vi "HCC Cluster Arrays ReadWrite.vi"(0 "Array Label":string(combo)="Aisle1", 1 "Write?":bool, 5 "configuration file path":path=path "C:/data/Wilt Backup.ini", 7 "Array Dryers In":T1[](array[typedef]) {"Unit Type" items=["", "Viper", "Hawk", "Other"]; "Current" format="%.2f"; "Day Cycle Count" format="%04d"}, 11 "error in (no error)":errorcluster) -> (8 "Array Dryers Out":T1[](array[typedef]) {"Unit Type" items=["", "Viper", "Hawk", "Other"]; "Current" format="%.2f"; "Day Cycle Count" format="%04d"}, 15 "error out":errorcluster)   [LabVIEW 2012]
uses:
  <vilib>/Utility/VariantDataType/Type.ctl
  Nufi/Newfi LDN/Washer.ctl
  Nufi/Newfi LDN/Washer Details.ctl
  Nufi/Newfi LDN/Unit Type.ctl
  <vilib>/Utility/config.llb/Write Key (Double).vi
  <vilib>/Utility/config.llb/Write Key (String).vi
  <vilib>/Utility/config.llb/Write Key (Path).vi
  <vilib>/Utility/config.llb/Write Key (I32).vi
  <vilib>/Utility/config.llb/Write Key (U32).vi
  <vilib>/Utility/config.llb/Write Key (Boolean).vi
  <vilib>/Utility/config.llb/Read Key (Double).vi
  <vilib>/Utility/config.llb/Read Key (String).vi
  <vilib>/Utility/config.llb/Read Key (Path).vi
  <vilib>/Utility/config.llb/Read Key (I32).vi
  <vilib>/Utility/config.llb/Read Key (U32).vi
  <vilib>/Utility/config.llb/Read Key (Boolean).vi
  <vilib>/Utility/config.llb/NI_LVConfig.lvlib
  <vilib>/Utility/VariantDataType/VariantType.lvlib
panel:
  out "Label.Text 2":string
  out "Local Control?":bool
  in  "Array Dryers Display":T1[](array[typedef]) {"Unit Type" items=["", "Viper", "Hawk", "Other"]; "Current" format="%.2f"; "Day Cycle Count" format="%04d"}
  out "value":string
  in  "Dryer Variable":T1 {"Unit Type" items=["", "Viper", "Hawk", "Other"]; "Current" format="%.2f"; "Day Cycle Count" format="%04d"}
  out "String array out":string="[1,23-2-3]\n[4-3,22-2]\n[3-4,01-8]\n[0-7-6,66]"
  out "Label.Text":string
  out "Type Enum":T4
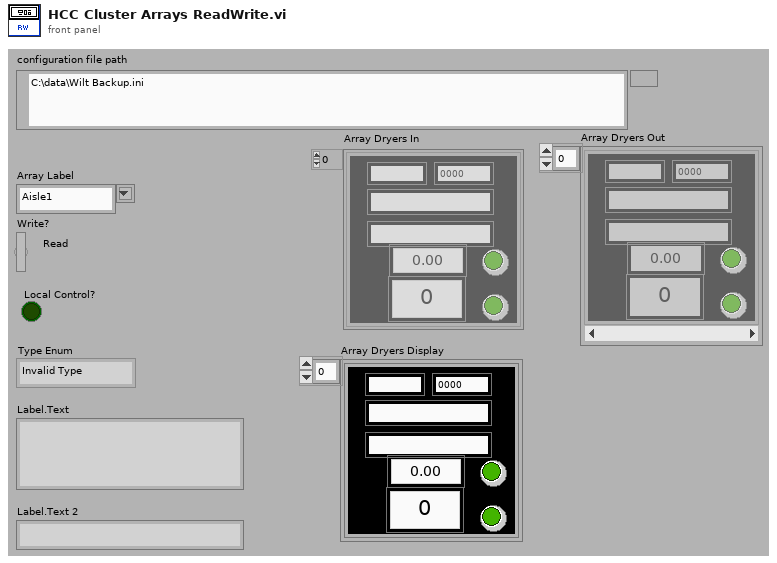
[diagram p1: front panel]
types:
  T1 = typedef "Washer.ctl" = cluster{"Serial Number":string, "Day Cycle Count":i32, "Station Label":string, "Status Color":u32, "Current Run Start Time":dbl, "Audit Alert":bool, "Washer Details":T2, "Board ID":string, "Boolean":bool, "RPM":u32, "Current":dbl, "Current Path":path, "Saving":bool, "Unit Type":T3}
  T2 = typedef "Washer Details.ctl" = cluster{"Cycle Count":string, "Status":string, "Notes":string, "Lab ID":string, "Total Time On":string, "TR Number":string}
  T3 = typedef "Unit Type.ctl" = u32
  T4 = typedef "VariantType.lvlib/Type.ctl" = enum8{"Invalid Type", "Void", "I8", "I16", "I32", "I64", "U8", "U16", "U32", "U64", "Single Float", "Double Float", "Extended Float", "Single Complex", "Double Complex", "Extended Complex", "Enum U8", "Enum U16", "Enum U32", "Enum U64", "Single Float With Unit", "Double Float With Unit", "Extended Float With Unit", "Single Complex with Unit", "Double Complex with Unit", "Extended Complex with Unit", "Boolean", "String", "Path", "Picture", "Tag", "Array", "Cluster", "Variant", "LV Variant", "Waveform", "Timestamp", "Digital Waveform", "Digital Data", "ExpressData", "Refnum", "External Data", "VI", "Poly VI", "LabVIEW Class Instance", "Fixed Point"}
  T5 = typedef "NI_LVConfig.lvlib/Config Data RefNum.ctl" = refnum<k1>
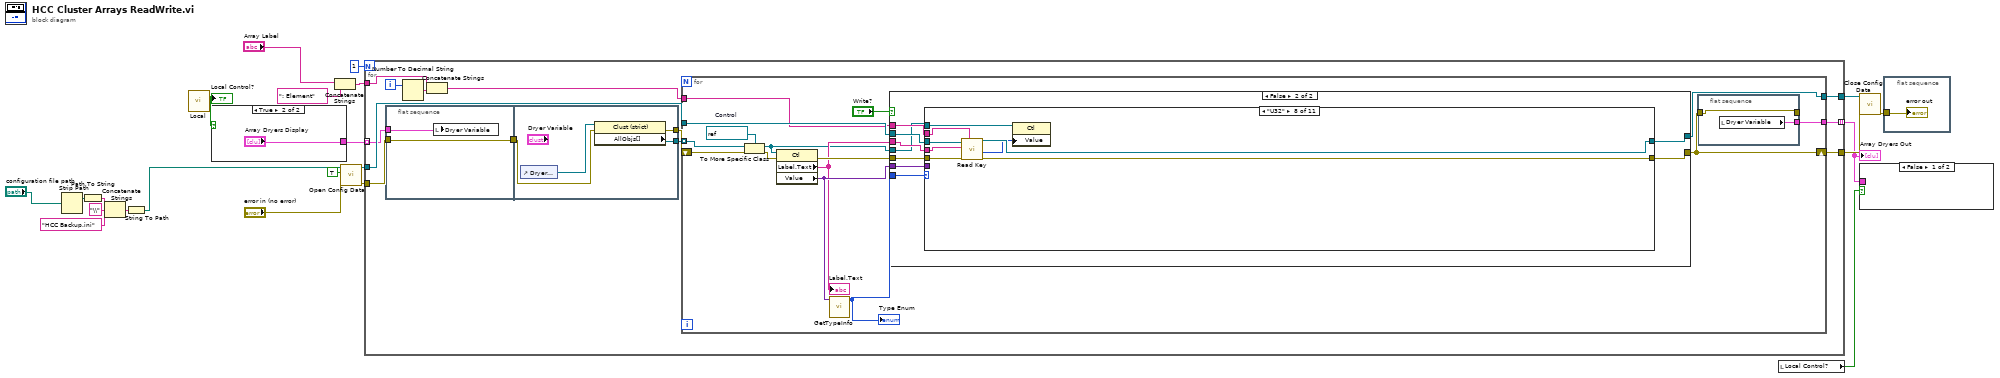
[diagram p0: block diagram]
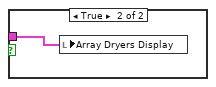
[diagram p2: hidden frame]
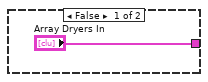
[diagram p3: hidden frame]
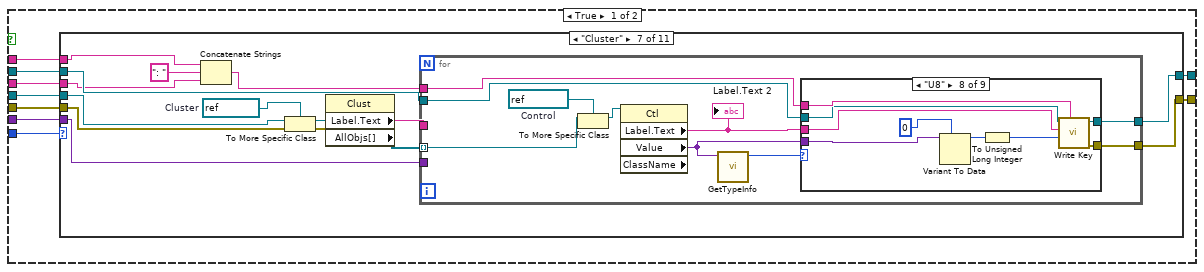
[diagram p4: hidden frame]
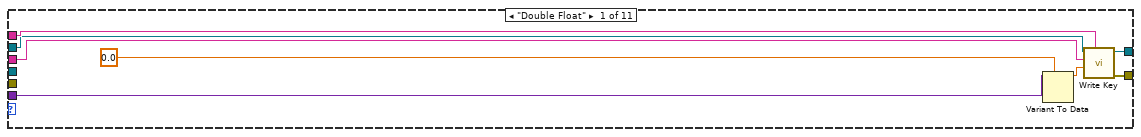
[diagram p5: hidden frame]
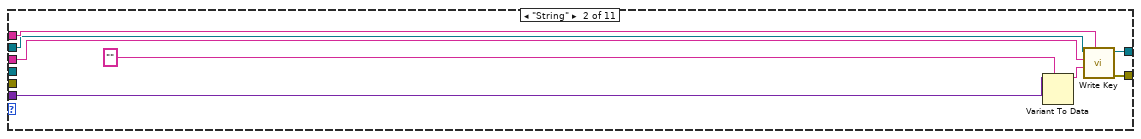
[diagram p6: hidden frame]
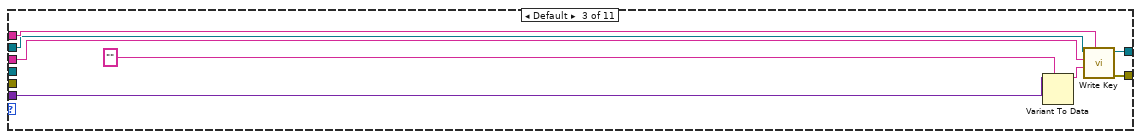
[diagram p7: hidden frame]
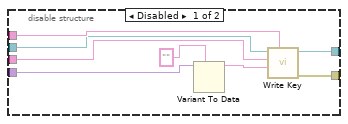
[diagram p9: hidden frame]
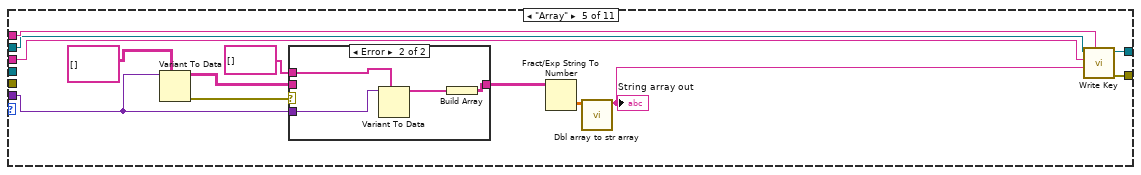
[diagram p10: hidden frame]
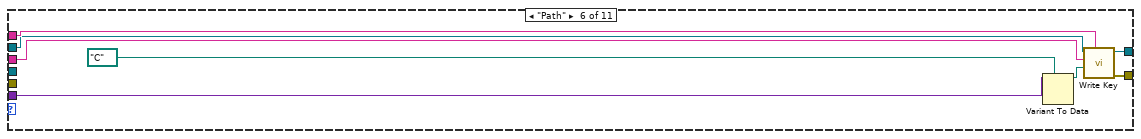
[diagram p12: hidden frame]
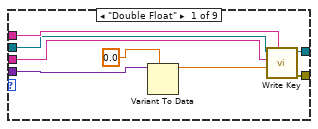
[diagram p13: hidden frame]
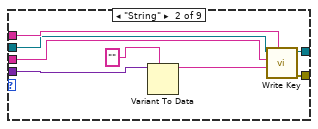
[diagram p14: hidden frame]
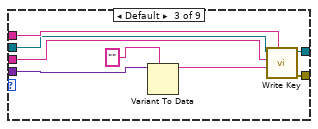
[diagram p15: hidden frame]
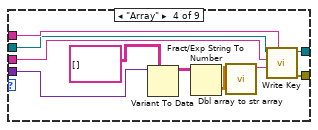
[diagram p16: hidden frame]
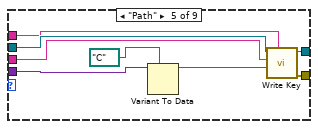
[diagram p17: hidden frame]
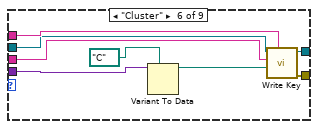
[diagram p18: hidden frame]
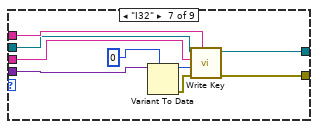
[diagram p19: hidden frame]
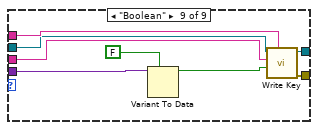
[diagram p20: hidden frame]
diagram:
  n1 = Strip Path(path="configuration file path") -> (stripped path=w5:path)  [unwired: 1 out]
  n2 = Path To String(path=w5) -> (string=w4:string)
  n3 = Concatenate Strings(w4, "\\" ("string"), "HCC Backup.ini" ("string")) -> (w8:string)
  n4 = String To Path(string=w8) -> (path=w2:path)
  n5 = call "Local.vi"() -> ("Local?"=w9:bool)  [unwired: 11 in]
  "Local Control?" <- w9
  n6 = case shown="True" w9 {
    tunnel: ["Array Dryers In" "Array Dryers Display"] -> w11
    frame False {
    }
    frame True {
    }
  }
  n7 = Concatenate Strings("Array Label", ": Element" ("string")) -> (w16:string)
  n8 = call <vilib>:"Open Config Data.vi"("error in (no error)"="error in (no error)", "create file if necessary (T)"=TRUE, "configuration file path"=w2) -> ("error out"=w19:errorcluster, "refnum"=w21:T5)  [unwired: 6 in, 1 out]
  n9 = for {
    N: 1 -> [_]
    tunnel: w19 -> [w36]
    tunnel: w11 -> [w32] mode=indexing
    tunnel: w21 -> [w34]
    tunnel: w16 -> [w30]
    tunnel: [w27] -> w14
    tunnel: [w26] -> w13
    tunnel: [w25] -> w12 mode=indexing
    i -> [w28]
    n10 = flat-sequence {
      tunnel: w36 -> [w39]
      tunnel: [w39] -> w33
      tunnel: w32 -> [w38]
      tunnel: [w43] -> w37
      tunnel: [w41] -> w35
      tunnel: w33 -> [w42]
      frame #0 {
        n11 = local write "Dryer Variable"(w38) -> ()
      }
      frame #1 {
        n12 = control-ref of="Dryer Variable"() -> (w40:refnum<vi>)
        n13 = property class="Clust (strict)"(reference=w40, error in=w42) -> (error out=w41:errorcluster, "AllObjs[]"=w43:refnum<vi>[])  [unwired: 1 out]
      }
    }
    n14 = Number To Decimal String(number=w28) -> (decimal integer string=w31:string)  [unwired: 1 in]
    n15 = Concatenate Strings(w30, w31) -> (w29:string)
    n16 = for {
      tunnel: w37 -> [w58] mode=indexing
      tunnel: w34 -> [w56]
      tunnel: [w55] -> w26
      shift-right: [w46] -> w27
      shift-left: w35 -> [w54]
      tunnel: w29 -> [w47]
      tunnel: [w45] -> w25
      w57 = refnum<vi> refnum  # Control
      n17 = To More Specific Class(target class=w57, reference=w58, error in=w54) -> (specific class reference=w44:refnum<vi>, error out=w49:errorcluster)
      n18 = property class="Ctl"(reference=w44, error in=w49) -> (error out=w50:errorcluster, "Label.Text"=w48:string, "Value"=w51:variant)  [unwired: 1 out]
      "Label.Text" <- w48
      n19 = call <vilib>:"GetTypeInfo.vi"("Variant"=w51) -> ("Type Enum"=w52:T4)  [unwired: 6 in, 4 out]
      "Type Enum" <- w52
      n20 = case shown="False" "Write?" {
        tunnel: w47 -> [w69 w276]
        tunnel: w48 -> [w68 w275]
        tunnel: w51 -> [w67 w268]
        tunnel: w56 -> [w66 w274]
        tunnel: [w65 w273] -> w46
        tunnel: [w64 w272] -> w55
        tunnel: w44 -> [w61 w271]
        tunnel: w52 -> [w63 w270]
        tunnel: w50 -> [w62 w269]
        frame True {
          n21 = case shown="\"Cluster\"" w63 {
            tunnel: w69 -> [w77 w85 w93 w99 w120 w133 w136 w242 w250 w259 w267]
            tunnel: w68 -> [w76 w84 w92 w98 w119 w132 w135 w241 w249 w258 w266]
            tunnel: w67 -> [w75 w83 w91 w97 w109 w131 w144 w240 w248 w257 w265]
            tunnel: w66 -> [w74 w82 w90 w96 w118 w130 w138 w239 w247 w256 w264]
            tunnel: [w73 w81 w89 w95 w117 w129 w142 w238 w246 w255 w263] -> w65
            tunnel: [w72 w80 w88 w94 w116 w128 w143 w237 w245 w254 w262] -> w64
            tunnel: w62 -> [_ _ _ _ _ _ w145 _ _ _ _]
            tunnel: w61 -> [_ _ _ _ _ _ w140 _ _ _ _]
            frame "Double Float" {
              n22 = Variant To Data(type=0.0, Variant=w75) -> (data=w71:dbl)  [unwired: 1 in, 1 out]
              n23 = call-poly <vilib>:"Write Key.vi"("section"=w77, "value"=w71, "key"=w76, "refnum"=w74) -> ("error out"=w73:errorcluster, "refnum out"=w72:T5)  [unwired: 5 in, 1 out]
            }
            frame "String" {
              n24 = Variant To Data(type="" ("Label.Text"), Variant=w83) -> (data=w79:string)  [unwired: 1 in, 1 out]
              n25 = call-poly <vilib>:"Write Key.vi"("section"=w85, "value"=w79, "key"=w84, "refnum"=w82) -> ("error out"=w81:errorcluster, "refnum out"=w80:T5)  [unwired: 5 in, 1 out]
            }
            frame Default {
              n26 = Variant To Data(type="" ("Label.Text"), Variant=w91) -> (data=w87:string)  [unwired: 1 in, 1 out]
              n27 = call-poly <vilib>:"Write Key.vi"("section"=w93, "value"=w87, "key"=w92, "refnum"=w90) -> ("error out"=w89:errorcluster, "refnum out"=w88:T5)  [unwired: 5 in, 1 out]
            }
            frame "Void" {
              n28 = disable-structure shown="Enabled" {
                disable-tunnel: w99 -> [w107 _]
                disable-tunnel: w98 -> [w106 _]
                disable-tunnel: w97 -> [w105 _]
                disable-tunnel: w96 -> [w104 _]
                disable-tunnel: [w103 _] -> w95
                disable-tunnel: [w102 _] -> w94
                frame Disabled {
                  n29 = Variant To Data(type="" ("Label.Text"), Variant=w105) -> (data=w101:string)  [unwired: 1 in, 1 out]
                  n30 = call-poly <vilib>:"Write Key.vi"("section"=w107, "value"=w101, "key"=w106, "refnum"=w104) -> ("error out"=w103:errorcluster, "refnum out"=w102:T5)  [unwired: 5 in, 1 out]
                }
                frame Enabled {
                }
              }
            }
            frame "Array" {
              n31 = Variant To Data(type=string[][] [], Variant=w109) -> (data=w111:string[][], error out=w112:errorcluster)  [unwired: 1 in]
              n32 = case shown="Error" w112 {
                tunnel: [w121 w122] -> w110
                tunnel: w111 -> [w121 _]
                tunnel: w109 -> [_ w125]
                tunnel: string[] [] -> [_ w124]
                frame No Error {
                }
                frame Error {
                  n33 = Variant To Data(type=w124, Variant=w125) -> (data=w123:string[])  [unwired: 1 in, 1 out]
                  n34 = Build Array(w123) -> (w122:string[][])
                }
              }
              n35 = Fract/Exp String To Number(string=w110) -> (number=w114:dbl[][])  [unwired: 3 in, 1 out]
              n36 = call "Dbl array to str array.vi"("Array in"=w114) -> ("String array out"=w113:string)  [unwired: 9 in, 1 out]
              "String array out" <- w113
              n37 = call-poly <vilib>:"Write Key.vi"("section"=w120, "value"=w113, "key"=w119, "refnum"=w118) -> ("error out"=w117:errorcluster, "refnum out"=w116:T5)  [unwired: 5 in, 1 out]
            }
            frame "Path" {
              n38 = Variant To Data(type=path "C:/" ("configuration file path 2"), Variant=w131) -> (data=w127:path)  [unwired: 1 in, 1 out]
              n39 = call-poly <vilib>:"Write Key.vi"("section"=w133, "value"=w127, "key"=w132, "refnum"=w130) -> ("error out"=w129:errorcluster, "refnum out"=w128:T5)  [unwired: 5 in, 1 out]
            }
            frame "Cluster" {
              w148 = refnum<vi> refnum  # Cluster
              n40 = Concatenate Strings(w136, ": " ("string"), w135) -> (w137:string)
              n41 = To More Specific Class(target class=w148, reference=w140, error in=w145) -> (specific class reference=w147:refnum<vi>, error out=w146:errorcluster)
              n42 = property class="Clust"(reference=w147, error in=w146) -> ("Label.Text"=w141:string, "AllObjs[]"=w139:refnum<vi>[])  [unwired: 2 out]
              n43 = for {
                tunnel: w144 -> [_]
                tunnel: w137 -> [w158]
                tunnel: w139 -> [w153] mode=indexing
                tunnel: [w157] -> w143
                tunnel: [w156] -> w142
                tunnel: w141 -> [_]
                tunnel: w138 -> [w152]
                w155 = refnum<vi> refnum  # Control
                n44 = To More Specific Class(target class=w155, reference=w153) -> (specific class reference=w154:refnum<vi>)  [unwired: 1 in, 1 out]
                n45 = property class="Ctl" props=["Label", "Text", "Value", "ClassName"](reference=w154) -> ("Label.Text"=w149:string, "Value"=w150:variant)  [unwired: 1 in, 3 out]
                "Label.Text 2" <- w149
                n46 = call <vilib>:"GetTypeInfo.vi"("Variant"=w150) -> ("Type Enum"=w151:T4)  [unwired: 6 in, 4 out]
                n47 = case shown="\"U8\"" w151 {
                  tunnel: w158 -> [w166 w174 w182 w192 w194 w208 w217 w226 w234]
                  tunnel: w149 -> [w165 w173 w175 w191 w193 w207 w216 w225 w233]
                  tunnel: w150 -> [w164 w172 w181 w190 w200 w206 w215 w224 w232]
                  tunnel: w152 -> [w159 w167 w176 w183 w195 w201 w209 w218 w227]
                  tunnel: [w163 w171 w180 w189 w199 w205 w214 w223 w231] -> w156
                  tunnel: [w162 w170 w179 w188 w198 w204 w213 w222 w230] -> w157
                  frame "Double Float" {
                    n48 = Variant To Data(type=0.0, Variant=w164) -> (data=w160:dbl)  [unwired: 1 in, 1 out]
                    n49 = call-poly <vilib>:"Write Key.vi"("section"=w166, "value"=w160, "key"=w165, "refnum"=w159) -> ("error out"=w163:errorcluster, "refnum out"=w162:T5)  [unwired: 5 in, 1 out]
                  }
                  frame "String" {
                    n50 = Variant To Data(type="" ("Label.Text"), Variant=w172) -> (data=w168:string)  [unwired: 1 in, 1 out]
                    n51 = call-poly <vilib>:"Write Key.vi"("section"=w174, "value"=w168, "key"=w173, "refnum"=w167) -> ("error out"=w171:errorcluster, "refnum out"=w170:T5)  [unwired: 5 in, 1 out]
                  }
                  frame Default {
                    n52 = Variant To Data(type="" ("Label.Text"), Variant=w181) -> (data=w177:string)  [unwired: 1 in, 1 out]
                    n53 = call-poly <vilib>:"Write Key.vi"("section"=w182, "value"=w177, "key"=w175, "refnum"=w176) -> ("error out"=w180:errorcluster, "refnum out"=w179:T5)  [unwired: 5 in, 1 out]
                  }
                  frame "Array" {
                    n54 = Variant To Data(type=string[][] [], Variant=w190) -> (data=w186:string[][])  [unwired: 1 in, 1 out]
                    n55 = Fract/Exp String To Number(string=w186) -> (number=w185:dbl[][])  [unwired: 3 in, 1 out]
                    n56 = call "Dbl array to str array.vi"("Array in"=w185) -> ("String array out"=w184:string)  [unwired: 9 in, 1 out]
                    n57 = call-poly <vilib>:"Write Key.vi"("section"=w192, "value"=w184, "key"=w191, "refnum"=w183) -> ("error out"=w189:errorcluster, "refnum out"=w188:T5)  [unwired: 5 in, 1 out]
                  }
                  frame "Path" {
                    n58 = Variant To Data(type=path "C:/" ("configuration file path 2"), Variant=w200) -> (data=w196:path)  [unwired: 1 in, 1 out]
                    n59 = call-poly <vilib>:"Write Key.vi"("section"=w194, "value"=w196, "key"=w193, "refnum"=w195) -> ("error out"=w199:errorcluster, "refnum out"=w198:T5)  [unwired: 5 in, 1 out]
                  }
                  frame "Cluster" {
                    n60 = Variant To Data(type=path "C:/" ("configuration file path 2"), Variant=w206) -> (data=w202:path)  [unwired: 1 in, 1 out]
                    n61 = call-poly <vilib>:"Write Key.vi"("section"=w208, "value"=w202, "key"=w207, "refnum"=w201) -> ("error out"=w205:errorcluster, "refnum out"=w204:T5)  [unwired: 5 in, 1 out]
                  }
                  frame "I32" {
                    n62 = Variant To Data(type=0, Variant=w215) -> (data=w210:i32, error out=w211:errorcluster)  [unwired: 1 in]
                    n63 = call-poly <vilib>:"Write Key.vi"("section"=w217, "error in (no error)"=w211, "value"=w210, "key"=w216, "refnum"=w209) -> ("error out"=w214:errorcluster, "refnum out"=w213:T5)  [unwired: 4 in, 1 out]
                  }
                  frame "U8" {
                    n64 = Variant To Data(type=u8 0, Variant=w224) -> (data=w221:u8)  [unwired: 1 in, 1 out]
                    n65 = To Unsigned Long Integer(number=w221) -> (unsigned 32bit integer=w219:u32)
                    n66 = call-poly <vilib>:"Write Key.vi"("section"=w226, "value"=w219, "key"=w225, "refnum"=w218) -> ("error out"=w223:errorcluster, "refnum out"=w222:T5)  [unwired: 5 in, 1 out]
                  }
                  frame "Boolean" {
                    n67 = Variant To Data(type=FALSE ("Write? 2"), Variant=w232) -> (data=w229:bool)  [unwired: 1 in, 1 out]
                    n68 = call-poly <vilib>:"Write Key.vi"("section"=w234, "value"=w229, "key"=w233, "refnum"=w227) -> ("error out"=w231:errorcluster, "refnum out"=w230:T5)  [unwired: 5 in, 1 out]
                  }
                }
              }
            }
            frame "I32" {
              n69 = Variant To Data(type=0, Variant=w240) -> (data=w236:i32)  [unwired: 1 in, 1 out]
              n70 = call-poly <vilib>:"Write Key.vi"("section"=w242, "value"=w236, "key"=w241, "refnum"=w239) -> ("error out"=w238:errorcluster, "refnum out"=w237:T5)  [unwired: 5 in, 1 out]
            }
            frame "U32" {
              n71 = Variant To Data(type=0, Variant=w248) -> (data=w244:i32)  [unwired: 1 in, 1 out]
              n72 = call-poly <vilib>:"Write Key.vi"("section"=w250, "value"=w244, "key"=w249, "refnum"=w247) -> ("error out"=w246:errorcluster, "refnum out"=w245:T5)  [unwired: 5 in, 1 out]
            }
            frame "U8" {
              n73 = Variant To Data(type=u8 0, Variant=w257) -> (data=w253:u8)  [unwired: 1 in, 1 out]
              n74 = To Unsigned Long Integer(number=w253) -> (unsigned 32bit integer=w251:u32)
              n75 = call-poly <vilib>:"Write Key.vi"("section"=w259, "value"=w251, "key"=w258, "refnum"=w256) -> ("error out"=w255:errorcluster, "refnum out"=w254:T5)  [unwired: 5 in, 1 out]
            }
            frame "Boolean" {
              n76 = Variant To Data(type=FALSE ("Write? 2"), Variant=w265) -> (data=w261:bool)  [unwired: 1 in, 1 out]
              n77 = call-poly <vilib>:"Write Key.vi"("section"=w267, "value"=w261, "key"=w266, "refnum"=w264) -> ("error out"=w263:errorcluster, "refnum out"=w262:T5)  [unwired: 5 in, 1 out]
            }
          }
        }
        frame False {
          n78 = case shown="\"U32\"" w270 {
            tunnel: w276 -> [w283 w299 w307 w318 w326 w342 w435 w443 w451 w459 w467]
            tunnel: w275 -> [w282 w298 w306 w317 w333 w338 w442 w450 w458 w466 w474]
            tunnel: w274 -> [w281 w297 w305 w316 w332 w337 w441 w449 w457 w465 w473]
            tunnel: [w280 w296 w304 w315 w331 w335 w440 w448 w456 w464 w472] -> w273
            tunnel: [w279 w295 w303 w314 w330 w336 w439 w447 w455 w463 w471] -> w272
            tunnel: w271 -> [w278 w293 w301 w309 w328 w339 w437 w445 w453 w461 w469]
            tunnel: w269 -> [w277 w292 w300 w313 w327 w340 w436 w444 w452 w460 w468]
            tunnel: w268 -> [_ _ _ _ _ w341 _ _ _ _ _]
            frame "Void" {
              n79 = disable-structure shown="Enabled" {
                disable-tunnel: w283 -> [w291 _]
                disable-tunnel: w282 -> [w290 _]
                disable-tunnel: w281 -> [w289 _]
                disable-tunnel: [w288 _] -> w280
                disable-tunnel: [w287 _] -> w279
                disable-tunnel: w278 -> [w285 _]
                disable-tunnel: w277 -> [w284 _]
                frame Disabled {
                  n80 = call-poly <vilib>:"Read Key.vi"("section"=w291, "error in (no error)"=w284, "key"=w290, "refnum"=w289) -> ("error out"=w288:errorcluster, "value"=w286:bool, "refnum out"=w287:T5)  [unwired: 4 in, 1 out]
                  n81 = property class="Ctl"(reference=w285, "Value"=w286) -> ()  [unwired: 1 in, 2 out]
                }
                frame Enabled {
                }
              }
            }
            frame "Double Float" {
              n82 = call-poly <vilib>:"Read Key.vi"("section"=w299, "error in (no error)"=w292, "key"=w298, "refnum"=w297) -> ("error out"=w296:errorcluster, "value"=w294:dbl, "refnum out"=w295:T5)  [unwired: 4 in, 1 out]
              n83 = property class="Ctl"(reference=w293, "Value"=w294) -> ()  [unwired: 1 in, 2 out]
            }
            frame "String" {
              n84 = call-poly <vilib>:"Read Key.vi"("section"=w307, "error in (no error)"=w300, "key"=w306, "refnum"=w305) -> ("error out"=w304:errorcluster, "value"=w302:string, "refnum out"=w303:T5)  [unwired: 4 in, 1 out]
              n85 = property class="Ctl"(reference=w301, "Value"=w302) -> ()  [unwired: 1 in, 2 out]
            }
            frame "Array" {
              n86 = call-poly <vilib>:"Read Key.vi"("section"=w318, "error in (no error)"=w313, "key"=w317, "refnum"=w316) -> ("error out"=w315:errorcluster, "value"=w312:string, "refnum out"=w314:T5)  [unwired: 4 in, 1 out]
              "value" <- w312
              n87 = call "Str array to dbl array.vi"("String array in"=w312) -> ("Double array out"=w311:dbl[][])  [unwired: 9 in, 1 out]
              n88 = Number To Fractional String(number=w311) -> (F-format string=w308:string[][])  [unwired: 3 in]
              n89 = property class="Ctl"(reference=w309, "Value"=w308) -> (error out=w310:errorcluster)  [unwired: 1 in, 1 out]
              n90 = case shown="Error" w310 {
                tunnel: w309 -> [_ w325]
                tunnel: w308 -> [_ w324]
                frame No Error {
                }
                frame Error {
                  n91 = Array Subset(array=w324, index (row)=0 ("index")) -> (w321:string[][])  [unwired: 3 in]
                  n92 = Array Size(array=w321) -> (size(s)=w320:i32[])
                  n93 = Multiply Array Elements(1:w320) -> (0:w319:i32)
                  n94 = Reshape Array(w321, w319) -> (w322:string[])
                  n95 = property class="Ctl"(reference=w325, "Value"=w322) -> ()  [unwired: 1 in, 2 out]
                }
              }
            }
            frame "Path" {
              n96 = call-poly <vilib>:"Read Key.vi"("section"=w326, "error in (no error)"=w327, "key"=w333, "refnum"=w332) -> ("error out"=w331:errorcluster, "value"=w329:path, "refnum out"=w330:T5)  [unwired: 4 in, 1 out]
              n97 = property class="Ctl"(reference=w328, "Value"=w329) -> ()  [unwired: 1 in, 2 out]
            }
            frame "Cluster" {
              w349 = refnum<vi> refnum  # Cluster
              n98 = Concatenate Strings(w342, ": " ("string"), w338) -> (w344:string)
              n99 = To More Specific Class(target class=w349, reference=w339, error in=w340) -> (specific class reference=w348:refnum<vi>, error out=w347:errorcluster)
              n100 = property class="Clust"(reference=w348, error in=w347) -> (error out=w334:errorcluster, "Label.Text"=w346:string, "AllObjs[]"=w345:refnum<vi>[])  [unwired: 1 out]
              n101 = for {
                tunnel: w341 -> [_]
                tunnel: w344 -> [w352]
                tunnel: w345 -> [w359] mode=indexing
                tunnel: [w351] -> w336
                tunnel: [w355] -> w335
                tunnel: w346 -> [_]
                tunnel: w337 -> [w354]
                tunnel: w334 -> [w356]
                w361 = refnum<vi> refnum  # Control
                n102 = To More Specific Class(target class=w361, reference=w359) -> (specific class reference=w360:refnum<vi>)  [unwired: 1 in, 1 out]
                n103 = property class="Ctl"(reference=w360) -> (reference out=w353:refnum<vi>, "Label.Text"=w357:string, "Value"=w358:variant)  [unwired: 1 in, 1 out]
                n104 = call <vilib>:"GetTypeInfo.vi"("Variant"=w358) -> ("Type Enum"=w350:T4)  [unwired: 6 in, 4 out]
                n105 = case shown="Default" w350 {
                  tunnel: w352 -> [w369 w377 w385 w394 w395 w403 w411 w419 w427]
                  tunnel: w357 -> [w368 w376 w384 w393 w402 w410 w418 w426 w434]
                  tunnel: w354 -> [w367 w375 w383 w392 w401 w409 w417 w425 w433]
                  tunnel: [w366 w374 w382 w391 w400 w408 w416 w424 w432] -> w355
                  tunnel: [w365 w373 w381 w390 w399 w407 w415 w423 w431] -> w351
                  tunnel: w353 -> [w363 w371 w379 w389 w397 w405 w413 w421 w429]
                  tunnel: w356 -> [w362 w370 w378 w388 w396 w404 w412 w420 w428]
                  frame "Void" {
                    n106 = call-poly <vilib>:"Read Key.vi"("section"=w369, "error in (no error)"=w362, "key"=w368, "refnum"=w367) -> ("error out"=w366:errorcluster, "value"=w364:string, "refnum out"=w365:T5)  [unwired: 4 in, 1 out]
                    n107 = property class="Ctl"(reference=w363, "Value"=w364) -> ()  [unwired: 1 in, 2 out]
                  }
                  frame "Double Float" {
                    n108 = call-poly <vilib>:"Read Key.vi"("section"=w377, "error in (no error)"=w370, "key"=w376, "refnum"=w375) -> ("error out"=w374:errorcluster, "value"=w372:dbl, "refnum out"=w373:T5)  [unwired: 4 in, 1 out]
                    n109 = property class="Ctl"(reference=w371, "Value"=w372) -> ()  [unwired: 1 in, 2 out]
                  }
                  frame "String" {
                    n110 = call-poly <vilib>:"Read Key.vi"("section"=w385, "error in (no error)"=w378, "key"=w384, "refnum"=w383) -> ("error out"=w382:errorcluster, "value"=w380:string, "refnum out"=w381:T5)  [unwired: 4 in, 1 out]
                    n111 = property class="Ctl"(reference=w379, "Value"=w380) -> ()  [unwired: 1 in, 2 out]
                  }
                  frame "Array" {
                    n112 = call-poly <vilib>:"Read Key.vi"("section"=w394, "error in (no error)"=w388, "key"=w393, "refnum"=w392) -> ("error out"=w391:errorcluster, "value"=w387:string, "refnum out"=w390:T5)  [unwired: 4 in, 1 out]
                    n113 = call "Str array to dbl array.vi"("String array in"=w387) -> ("Double array out"=w386:dbl[][])  [unwired: 9 in, 1 out]
                    n114 = property class="Ctl"(reference=w389, "Value"=w386) -> ()  [unwired: 1 in, 2 out]
                  }
                  frame "Path" {
                    n115 = call-poly <vilib>:"Read Key.vi"("section"=w395, "error in (no error)"=w396, "key"=w402, "refnum"=w401) -> ("error out"=w400:errorcluster, "value"=w398:path, "refnum out"=w399:T5)  [unwired: 4 in, 1 out]
                    n116 = property class="Ctl"(reference=w397, "Value"=w398) -> ()  [unwired: 1 in, 2 out]
                  }
                  frame "I32" {
                    n117 = call-poly <vilib>:"Read Key.vi"("section"=w403, "error in (no error)"=w404, "key"=w410, "refnum"=w409) -> ("error out"=w408:errorcluster, "value"=w406:i32, "refnum out"=w407:T5)  [unwired: 4 in, 1 out]
                    n118 = property class="Ctl"(reference=w405, "Value"=w406) -> ()  [unwired: 1 in, 2 out]
                  }
                  frame "U32" {
                    n119 = call-poly <vilib>:"Read Key.vi"("section"=w411, "error in (no error)"=w412, "key"=w418, "refnum"=w417) -> ("error out"=w416:errorcluster, "value"=w414:u32, "refnum out"=w415:T5)  [unwired: 4 in, 1 out]
                    n120 = property class="Ctl"(reference=w413, "Value"=w414) -> ()  [unwired: 1 in, 2 out]
                  }
                  frame Default {
                    n121 = call-poly <vilib>:"Read Key.vi"("section"=w419, "error in (no error)"=w420, "key"=w426, "refnum"=w425) -> ("error out"=w424:errorcluster, "value"=w422:bool, "refnum out"=w423:T5)  [unwired: 4 in, 1 out]
                    n122 = property class="Ctl"(reference=w421, "Value"=w422) -> ()  [unwired: 1 in, 2 out]
                  }
                  frame "Boolean" {
                    n123 = call-poly <vilib>:"Read Key.vi"("section"=w427, "error in (no error)"=w428, "key"=w434, "refnum"=w433) -> ("error out"=w432:errorcluster, "value"=w430:bool, "refnum out"=w431:T5)  [unwired: 4 in, 1 out]
                    n124 = property class="Ctl"(reference=w429, "Value"=w430) -> ()  [unwired: 1 in, 2 out]
                  }
                }
              }
            }
            frame "I32" {
              n125 = call-poly <vilib>:"Read Key.vi"("section"=w435, "error in (no error)"=w436, "key"=w442, "refnum"=w441) -> ("error out"=w440:errorcluster, "value"=w438:i32, "refnum out"=w439:T5)  [unwired: 4 in, 1 out]
              n126 = property class="Ctl"(reference=w437, "Value"=w438) -> ()  [unwired: 1 in, 2 out]
            }
            frame "U32" {
              n127 = call-poly <vilib>:"Read Key.vi"("section"=w443, "error in (no error)"=w444, "key"=w450, "refnum"=w449) -> ("error out"=w448:errorcluster, "value"=w446:u32, "refnum out"=w447:T5)  [unwired: 4 in, 1 out]
              n128 = property class="Ctl"(reference=w445, "Value"=w446) -> ()  [unwired: 1 in, 2 out]
            }
            frame "U8" {
              n129 = call-poly <vilib>:"Read Key.vi"("section"=w451, "error in (no error)"=w452, "key"=w458, "refnum"=w457) -> ("error out"=w456:errorcluster, "value"=w454:u32, "refnum out"=w455:T5)  [unwired: 4 in, 1 out]
              n130 = property class="Ctl"(reference=w453, "Value"=w454) -> ()  [unwired: 1 in, 2 out]
            }
            frame Default {
              n131 = call-poly <vilib>:"Read Key.vi"("section"=w459, "error in (no error)"=w460, "key"=w466, "refnum"=w465) -> ("error out"=w464:errorcluster, "value"=w462:string, "refnum out"=w463:T5)  [unwired: 4 in, 1 out]
              n132 = property class="Ctl"(reference=w461, "Value"=w462) -> ()  [unwired: 1 in, 2 out]
            }
            frame "Boolean" {
              n133 = call-poly <vilib>:"Read Key.vi"("section"=w467, "error in (no error)"=w468, "key"=w474, "refnum"=w473) -> ("error out"=w472:errorcluster, "value"=w470:bool, "refnum out"=w471:T5)  [unwired: 4 in, 1 out]
              n134 = property class="Ctl"(reference=w469, "Value"=w470) -> ()  [unwired: 1 in, 2 out]
            }
          }
        }
      }
      n135 = flat-sequence {
        tunnel: [w60] -> _
        tunnel: w46 -> [w60]
        tunnel: [w59] -> w45
        frame #0 {
          n136 = local read "Dryer Variable"() -> (w59:T1)
        }
      }
    }
  }
  "Array Dryers Out" <- w12
  n137 = local read "Local Control?"() -> (w10:bool)
  n138 = call <vilib>:"Close Config Data.vi"("error in (no error)"=w14, "refnum"=w13) -> ("error out"=w15:errorcluster)  [unwired: 8 in, 1 out]
  n139 = case shown="False" w10 {
    tunnel: w12 -> [_ w475]
    frame False {
    }
    frame True {
      n140 = local write "Array Dryers Display"(w475) -> ()
    }
  }
  n141 = flat-sequence {
    tunnel: w15 -> [w476]
    frame #0 {
      "error out" <- w476
    }
  }
